vi "Control Visible Toggle.vi"(6 "Mouse Position":T1 caption="鼠标位置", 7 "User VI Ref":refnum<vi> caption="用户VI引用", 8 "Is Multi-select?":bool caption="为多选？", 9 "Remaining Items":refnum<vi>[](array[refnum]) caption="剩余项", 10 "Affected Items":T8 caption="受影响的项", 11 "Menu Refnum":refnum<k9> caption="菜单引用句柄") -> (3 "Menu Items To Add":T2[](array[typedef]) caption="待添加菜单项")   [LabVIEW 2020]
doc: "该VI属于修改LabVIEW快捷菜单部分。这是创建快捷菜单时调用的生成VI。该VI为LabVIEW输入添加到菜单的快捷菜单项。"
uses:
  <resource>/plugins/PopupMenus/support/Checkmark Status.ctl
  <resource>/plugins/PopupMenus/support/Relative Position.ctl
  <resource>/plugins/PopupMenus/support/Position In Menu.ctl
  <resource>/plugins/PopupMenus/support/Transaction Control.ctl
  <resource>/plugins/PopupMenus/support/Shortcut Menu Item Definition.ctl
  <resource>/plugins/PopupMenus/support/Enabled Menu Item Status.ctl
  Control Visible Toggle.ctl
  <vilib>/Utility/miscctls.llb/LVPositionTypeDef.ctl
panel:
  # "弹出插件时必须遵循的规则：\n*该VI的文件名称必须与LLB的文件名称匹配－不同的只是文件扩展名。\n*VI必须禁用调试，否则它将作为插件被忽略。\n*所有菜单项的“标签后缀 + VI文件名”必须少于240个字符。\n*可从自定义类型断开连接“受影响的项”，从而加快插件的加载速度。存在该自定义类型的目的是使该VI和执行VI使用相同的类型。\n*除“受影响的项”之外，前面板上的其他所有控件都已锁定，以防被意外编辑。除“受影响的项”簇中的元素外，不要修改控件的类型或名称。\n*请参考即时帮助，了解每个控件的详细信息。"
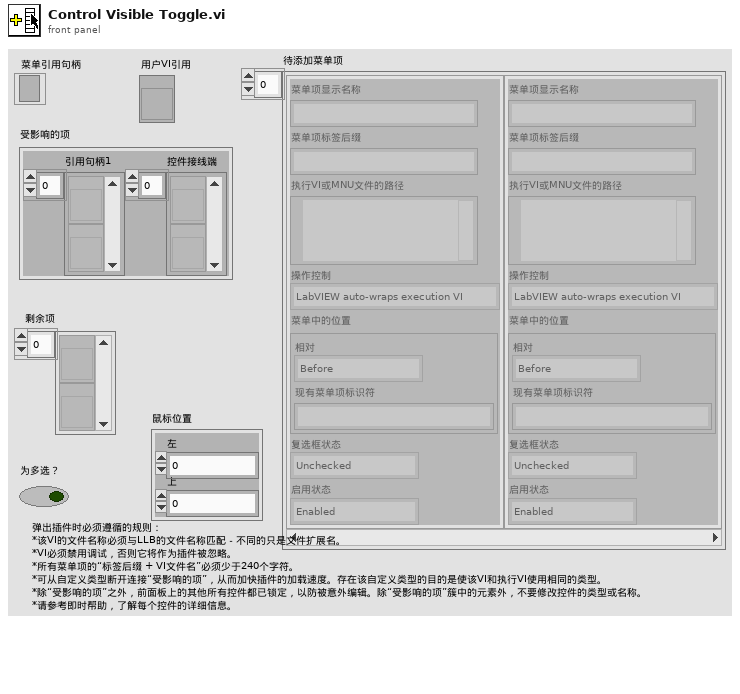
[diagram p1: front panel]
types:
  T1 = typedef "LVPositionTypeDef.ctl" = cluster{"Left":i32, "Top":i32}
  T2 = typedef "Shortcut Menu Item Definition.ctl" = cluster{"Menu Item Display Name":string, "Menu Item Tag Suffix":string, "Path To Execution VI or MNU":path, "Transaction Control":T3, "Position In Menu":T4, "Checkmark Status":T6, "Enabled Status":T7}
  T3 = typedef "Transaction Control.ctl" = enum8{"LabVIEW auto-wraps execution VI", "Execution VI will define if needed"}
  T4 = typedef "Position In Menu.ctl" = cluster{"Relative":T5, "Existing Item Tag":string}
  T5 = typedef "Relative Position.ctl" = enum8{"Before", "Instead of", "After", "Into Submenu"}
  T6 = typedef "Checkmark Status.ctl" = enum8{"Unchecked", "Checked"}
  T7 = typedef "Enabled Menu Item Status.ctl" = enum8{"Enabled", "Disabled"}
  T8 = typedef "Control Visible Toggle.ctl" = cluster{"Control":refnum<vi>[], "Control Term":refnum<vi>[]}
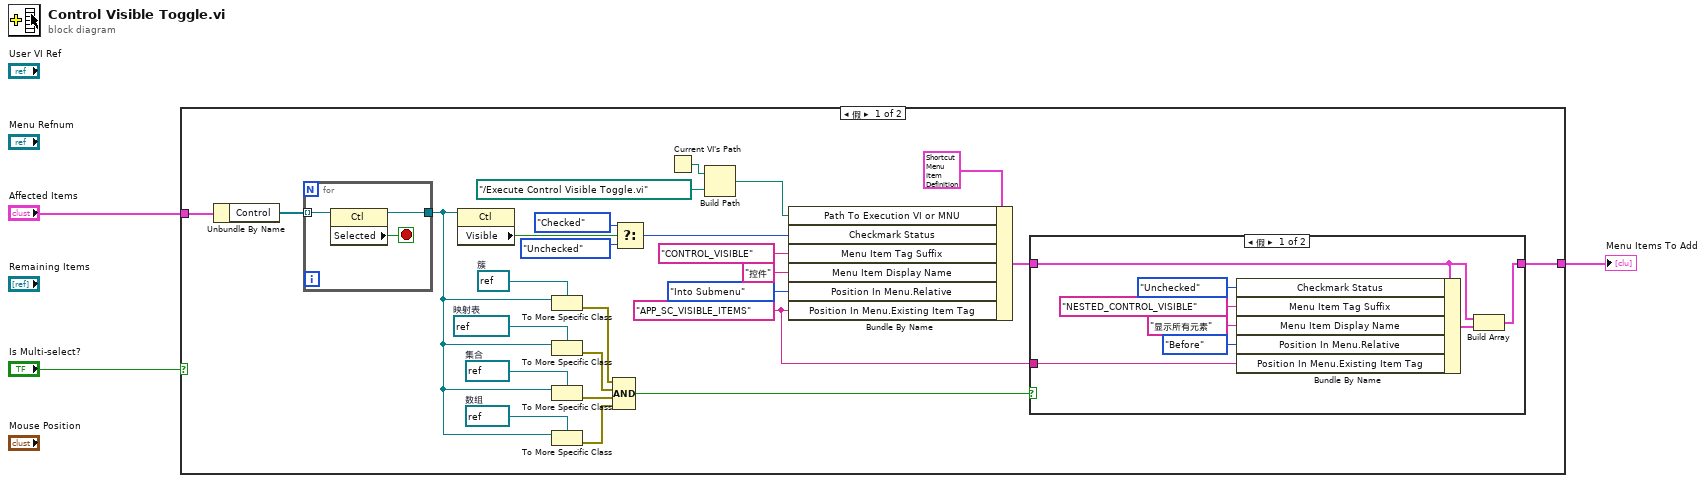
[diagram p0: block diagram]
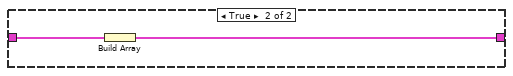
[diagram p2: hidden frame]
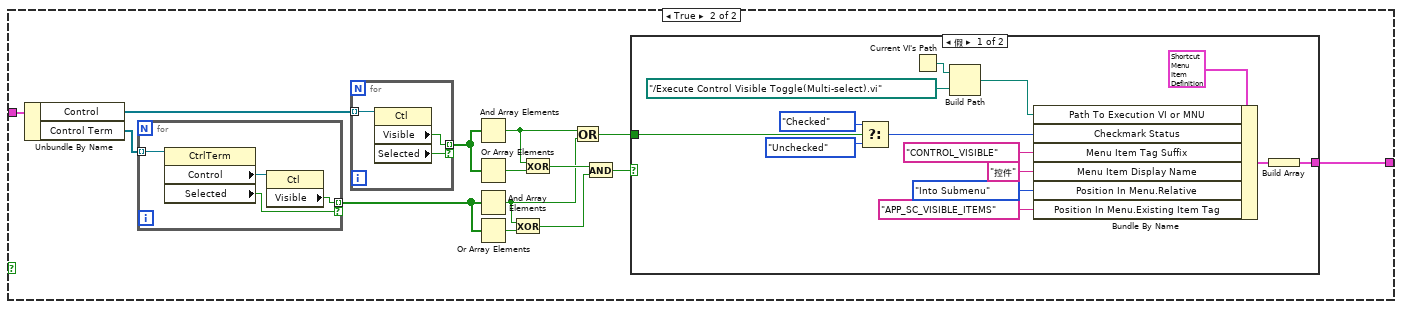
[diagram p3: hidden frame]
diagram:
  n1 = case shown="假" "Is Multi-select?" {
    tunnel: [w27 w54] -> w3
    tunnel: "Affected Items" -> [w25 w56]
    frame False {
      w12 = refnum<vi> refnum  # 数组
      w11 = refnum<vi> refnum  # 集合
      w10 = refnum<vi> refnum  # 映射表
      w9 = refnum<vi> refnum  # 簇
      w4 = "APP_SC_VISIBLE_ITEMS" ("项之后")
      n2 = Unbundle By Name(w25) -> ("Control"=w21:refnum<vi>[])
      n3 = for {
        tunnel: w21 -> [w42] mode=indexing
        tunnel: [w41] -> w8
        stop <- w40 stop-if-true
        n4 = property class="Ctl"(reference=w42) -> (reference out=w41:refnum<vi>, "Selected"=w40:bool)  [unwired: 1 in, 1 out]
      }
      n5 = property class="Ctl"(reference=w8) -> ("Visible"=w22:bool)  [unwired: 1 in, 2 out]
      n6 = To More Specific Class(target class=w9, reference=w8) -> (error out=w16:errorcluster)  [unwired: 1 in, 1 out]
      n7 = To More Specific Class(target class=w10, reference=w8) -> (error out=w15:errorcluster)  [unwired: 1 in, 1 out]
      n8 = To More Specific Class(target class=w11, reference=w8) -> (error out=w14:errorcluster)  [unwired: 1 in, 1 out]
      n9 = To More Specific Class(target class=w12, reference=w8) -> (error out=w13:errorcluster)  [unwired: 1 in, 1 out]
      n10 = Compound Arithmetic op=AND ("复合运算")(w16, w15, w14, w13) -> (w7:bool)
      n11 = Select(t=Checkmark_Status."Checked" ("Checkmark Status"), s=w22, f=Checkmark_Status."Unchecked" ("Checkmark Status")) -> (s? t:f=w20:T6)
      n12 = Current VI's Path() -> (path=w26:path)
      n13 = Build Path(base path=w26, name or relative path=path "../Execute Control Visible Toggle.vi" ("execute path")) -> (appended path=w6:path)
      n14 = Bundle By Name(cluster=T2 {"Menu Item Display Name"="", "Menu Item Tag Suffix"="", "Path To Execution VI or MNU"=path "", "Transaction Control"=enum."LabVIEW auto-wraps execution VI", "Position In Menu"={"Relative"=enum."Before", "Existing Item Tag"=""}, "Checkmark Status"=enum."Unchecked", "Enabled Status"=enum."Enabled"} ("Cluster"), "Path To Execution VI or MNU"=w6, "Checkmark Status"=w20, "Menu Item Tag Suffix"="CONTROL_VISIBLE" ("项之后"), "Menu Item Display Name"="控件" ("项名称"), "Position In Menu.Relative"=Relative_Position."Into Submenu", "Position In Menu.Existing Item Tag"=w4) -> (w19:T2)
      n15 = case shown="假" w7 {
        tunnel: [w37 w38] -> w27
        tunnel: w19 -> [w36 w39]
        tunnel: w4 -> [w31 _]
        frame False {
          n16 = Bundle By Name(cluster=w36, "Checkmark Status"=Checkmark_Status."Unchecked", "Menu Item Tag Suffix"="NESTED_CONTROL_VISIBLE" ("项之后"), "Menu Item Display Name"="显示所有元素" ("项名称"), "Position In Menu.Relative"=Relative_Position."Before", "Position In Menu.Existing Item Tag"=w31) -> (w34:T2)
          n17 = Build Array(w36, w34) -> (w37:T2[])
        }
        frame True {
          n18 = Build Array(w39) -> (w38:T2[])
        }
      }
    }
    frame True {
      n19 = Unbundle By Name(w56) -> ("Control"=w55:refnum<vi>[], "Control Term"=w51:refnum<vi>[])
      n20 = for {
        tunnel: w51 -> [w60] mode=indexing
        tunnel: [w57] -> w49 mode=indexing if=w59
        n21 = property class="CtrlTerm"(reference=w60) -> ("Control"=w58:refnum<vi>, "Selected"=w59:bool)  [unwired: 1 in, 2 out]
        n22 = property class="Ctl"(reference=w58) -> ("Visible"=w57:bool)  [unwired: 1 in, 2 out]
      }
      n23 = for {
        tunnel: w55 -> [w77] mode=indexing
        tunnel: [w76] -> w53 mode=indexing if=w75
        n24 = property class="Ctl"(reference=w77) -> ("Visible"=w76:bool, "Selected"=w75:bool)  [unwired: 1 in, 2 out]
      }
      n25 = And Array Elements(Boolean array=w53) -> (logical AND=w45:bool)
      n26 = Or Array Elements(Boolean array=w53) -> (logical OR=w52:bool)
      n27 = And Array Elements(Boolean array=w49) -> (logical AND=w44:bool)
      n28 = Or Array Elements(Boolean array=w49) -> (logical OR=w50:bool)
      n29 = Exclusive Or(1:w50, 2:w44) -> (0:w47:bool)
      n30 = Exclusive Or(1:w52, 2:w45) -> (0:w48:bool)
      n31 = Or(x=w45, y=w44) -> (x .or. y?=w43:bool)
      n32 = And(x=w48, y=w47) -> (x .and. y?=w46:bool)
      n33 = case shown="假" w46 {
        tunnel: [w62 _] -> w54
        tunnel: w43 -> [w61 _]
        frame False {
          n34 = Select(t=Checkmark_Status."Checked" ("Checkmark Status"), s=w61, f=Checkmark_Status."Unchecked" ("Checkmark Status")) -> (s? t:f=w69:T6)
          n35 = Current VI's Path() -> (path=w72:path)
          n36 = Build Path(base path=w72, name or relative path=path "../Execute Control Visible Toggle(Multi-select).vi" ("execute path")) -> (appended path=w66:path)
          n37 = Bundle By Name(cluster=T2 {"Menu Item Display Name"="", "Menu Item Tag Suffix"="", "Path To Execution VI or MNU"=path "", "Transaction Control"=enum."LabVIEW auto-wraps execution VI", "Position In Menu"={"Relative"=enum."Before", "Existing Item Tag"=""}, "Checkmark Status"=enum."Unchecked", "Enabled Status"=enum."Enabled"} ("Cluster"), "Path To Execution VI or MNU"=w66, "Checkmark Status"=w69, "Menu Item Tag Suffix"="CONTROL_VISIBLE" ("项之后"), "Menu Item Display Name"="控件" ("项名称"), "Position In Menu.Relative"=Relative_Position."Into Submenu", "Position In Menu.Existing Item Tag"="APP_SC_VISIBLE_ITEMS" ("项之后")) -> (w63:T2)
          n38 = Build Array(w63) -> (w62:T2[])
        }
        frame True {
        }
      }
    }
  }
  "Menu Items To Add" <- w3
